vi "ConfigDa.vi"(0 "Pump_1AI_1DO_2DI in":refnum<class "Engine_1DI_2DO.lvclass">, 11 "error in (no error)":errorcluster) -> (4 "Pump_1AI_1DO_2DI out":refnum<class "Engine_1DI_2DO.lvclass">, 15 "error out":errorcluster)   [LabVIEW 2019, in "Engine_1DI_2DO.lvclass"]
uses:
  Engine_1DI_2DO.lvclass
  D:/GIT H4000/H4000/src/Proccess_class/Proccess.lvclass
  Sig_DA_class/Sig_DA.lvclass
  Proccess_class/Proccess.lvclass/Proccess.ctl
  Engine_1DI_2DO.lvclass/Engine_1DI_2DO.ctl
  Proccess_class/Proccess.lvclass
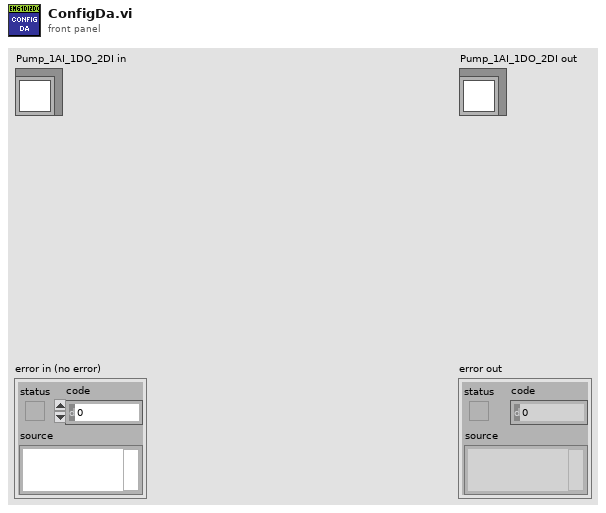
[diagram p1: front panel]
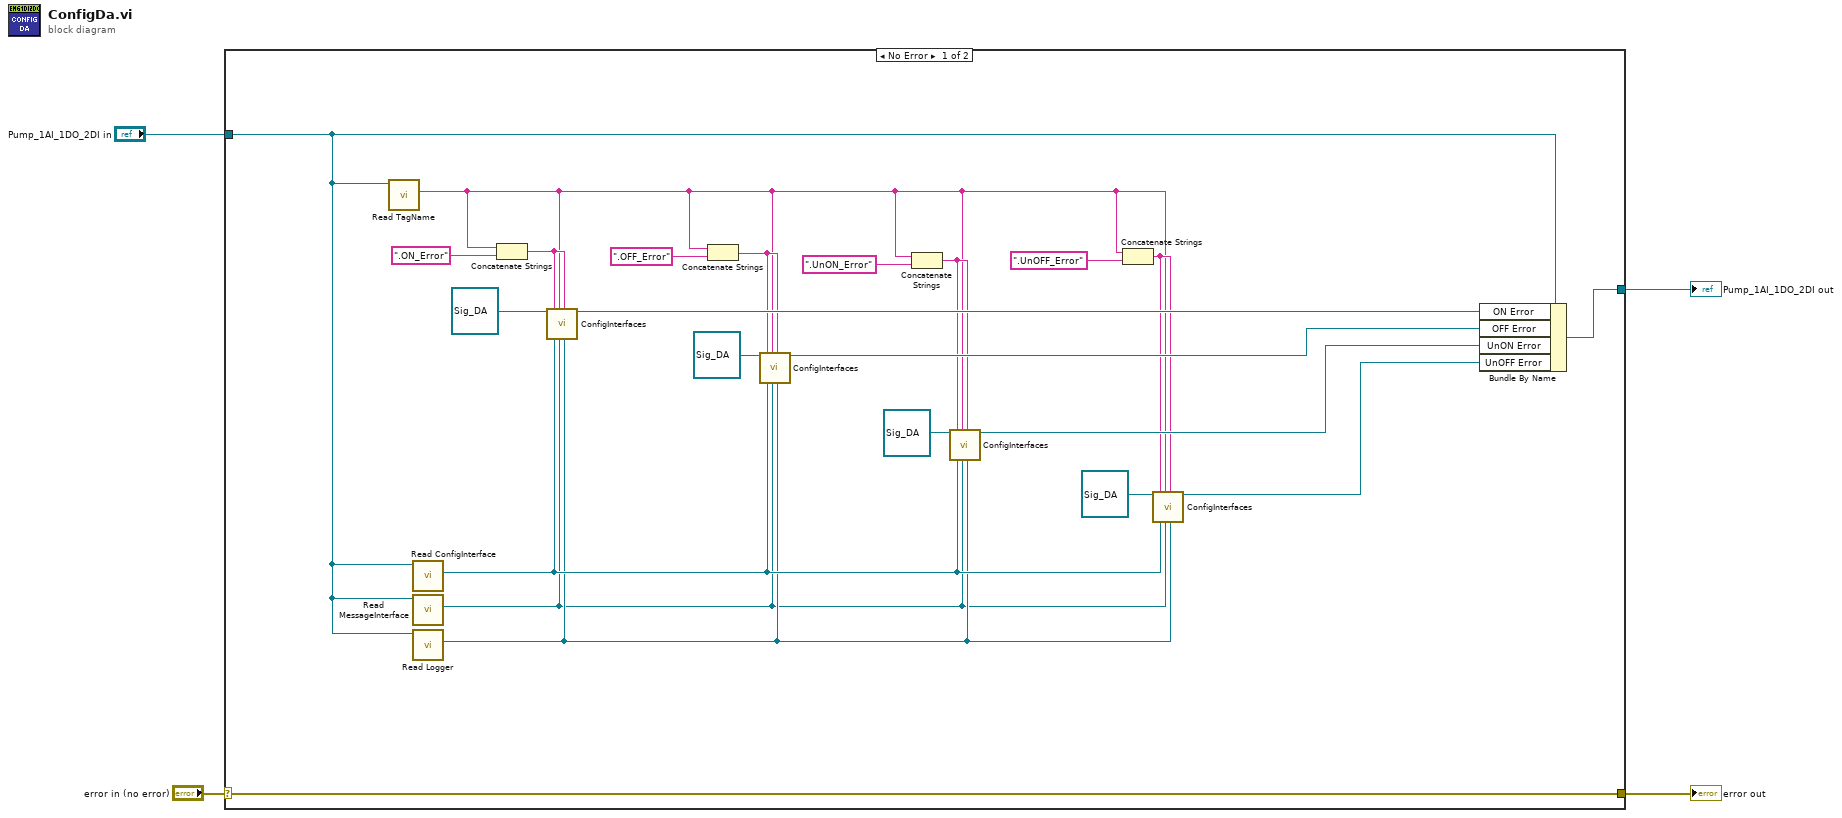
[diagram p0: block diagram]
diagram:
  n1 = case shown="No Error" "error in (no error)" {
    selector: "error in (no error)" -> [w27 w29]
    tunnel: [w27 w29] -> w3
    tunnel: [w26 w28] -> w1
    tunnel: "Pump_1AI_1DO_2DI in" -> [w14 w28]
    frame No Error {
      n2 = call "Read TagName.vi"("Proccess in"=w14) -> ("TagName"=w5:string)  [unwired: 9 in, 1 out]
      n3 = call "Read ConfigInterface.vi"("Proccess in"=w14) -> ("ConfigInterface"=w21:refnum<class "ConfigInterface.lvclass">)  [unwired: 9 in, 1 out]
      n4 = call "Read MessageInterface.vi"("Proccess in"=w14) -> ("MessageInterface"=w15:refnum<class "MessageInterface.lvclass">)  [unwired: 9 in, 1 out]
      n5 = call "Read Logger.vi"("Proccess in"=w14) -> ("Logger"=w16:refnum<class "Logger.lvclass">)  [unwired: 9 in, 1 out]
      n6 = Concatenate Strings(w5, ".ON_Error" ("string")) -> (w12:string)
      n7 = call "ConfigInterfaces.vi"("reference in"=refnum<class "Sig_DA.lvclass"> refnum ("Sig_DA"), "Name"=w12, "ConfigInterface"=w21, "ParentName"=w5, "MessageInterface"=w15, "Description"=w12, "Logger"=w16) -> ("reference out"=w25:refnum<class "Sig_DA.lvclass">)  [unwired: 11 in, 1 out]
      n8 = Concatenate Strings(w5, ".OFF_Error" ("string")) -> (w10:string)
      n9 = call "ConfigInterfaces.vi"("reference in"=refnum<class "Sig_DA.lvclass"> refnum ("Sig_DA"), "Name"=w10, "ConfigInterface"=w21, "ParentName"=w5, "MessageInterface"=w15, "Description"=w10, "Logger"=w16) -> ("reference out"=w24:refnum<class "Sig_DA.lvclass">)  [unwired: 11 in, 1 out]
      n10 = Concatenate Strings(w5, ".UnON_Error" ("string")) -> (w8:string)
      n11 = call "ConfigInterfaces.vi"("reference in"=refnum<class "Sig_DA.lvclass"> refnum ("Sig_DA"), "Name"=w8, "ConfigInterface"=w21, "ParentName"=w5, "MessageInterface"=w15, "Description"=w8, "Logger"=w16) -> ("reference out"=w23:refnum<class "Sig_DA.lvclass">)  [unwired: 11 in, 1 out]
      n12 = Concatenate Strings(w5, ".UnOFF_Error" ("string")) -> (w6:string)
      n13 = call "ConfigInterfaces.vi"("reference in"=refnum<class "Sig_DA.lvclass"> refnum ("Sig_DA"), "Name"=w6, "ConfigInterface"=w21, "ParentName"=w5, "MessageInterface"=w15, "Description"=w6, "Logger"=w16) -> ("reference out"=w22:refnum<class "Sig_DA.lvclass">)  [unwired: 11 in, 1 out]
      n14 = Bundle By Name(cluster=w14, "ON Error"=w25, "OFF Error"=w24, "UnON Error"=w23, "UnOFF Error"=w22) -> (w26:refnum<class "Engine_1DI_2DO.lvclass">)
    }
    frame Error {
    }
  }
  "error out" <- w3
  "Pump_1AI_1DO_2DI out" <- w1
